vi "GraphSettings(SubVI).vi"(8 "Error In":errorcluster, 10 "XYGraph Refnum":refnum<vi>, 11 "Cluster in":refnum<vi>) -> (0 "Error Out":errorcluster)   [LabVIEW 2018]
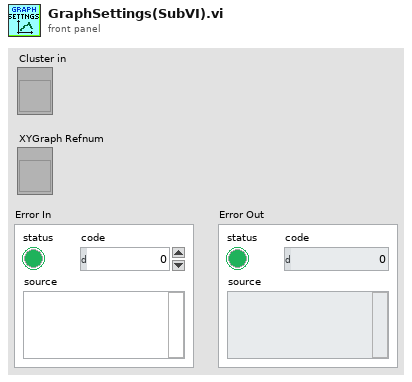
[diagram p1: front panel]
types:
  T1 = typedef "Graph settings.ctl" = cluster{"Axis X Min":dbl, "Axis X Name":string, "Axis X Max":dbl, "Axis Y Min":dbl, " Axis Y Name":string, "Axis Y Max":dbl, "Autoscale":enum16{"Yes", "No", "Only Oy", "Only Ox"}, "Choice Line":dbl}
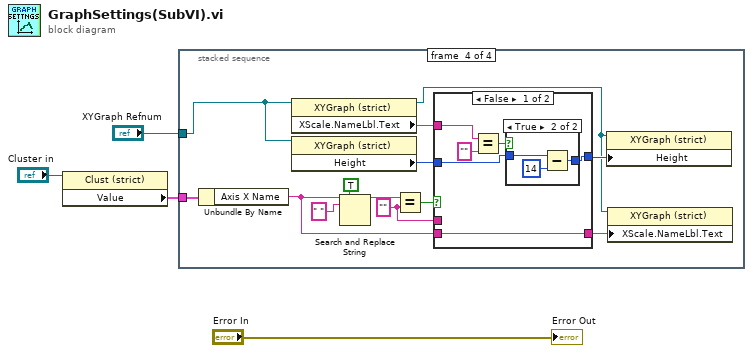
[diagram p0: block diagram]
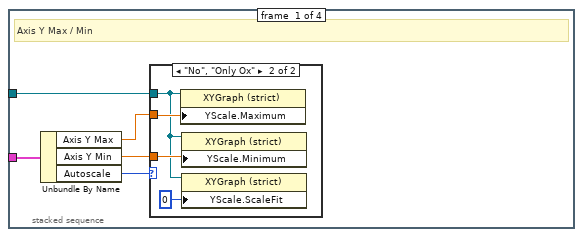
[diagram p2: hidden frame]
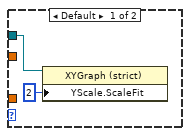
[diagram p3: hidden frame]
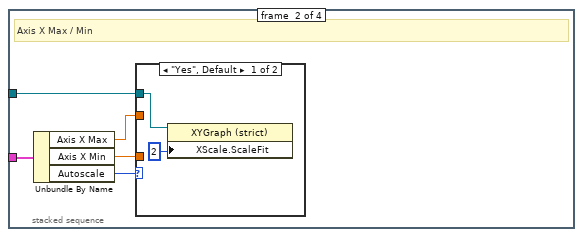
[diagram p4: hidden frame]
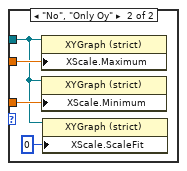
[diagram p5: hidden frame]
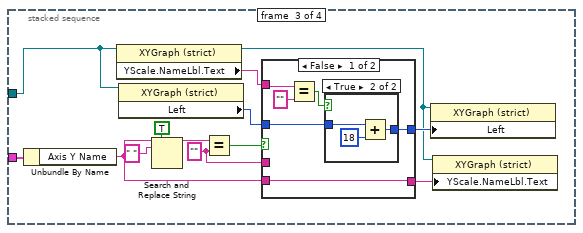
[diagram p6: hidden frame]
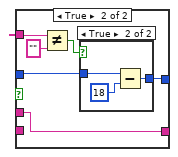
[diagram p8: hidden frame]
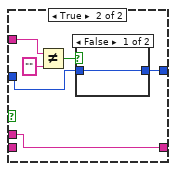
[diagram p11: hidden frame]
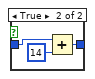
[diagram p12: hidden frame]
diagram:
  n1 = property on="Property Node" class="Clust (strict)"(reference="Cluster in") -> ("Value"=w4:T1)  [unwired: 1 in, 2 out]
  n2 = stacked-sequence {
    tunnel: w4 -> [w9 w20 w30 w63]
    tunnel: "XYGraph Refnum" -> [w5 w16 w28 w61]
    frame #0 {
      # "Axis Y Max / Min"
      n3 = Unbundle By Name(w9) -> ("Axis Y Max"=w8:dbl, "Axis Y Min"=w7:dbl, "Autoscale"=w6:enum16{"Yes", "No", "Only Oy", "Only Ox"})
      n4 = case shown="\"No\", \"Only Ox\"" w6 {
        tunnel: w8 -> [_ w15]
        tunnel: w7 -> [_ w14]
        tunnel: w5 -> [w10 w12]
        frame Default {
          n5 = property on="Property Node" class="XYGraph (strict)"(reference=w10, "YScale.ScaleFit"=u8 2 ("Y Scale.Scale Fit")) -> ()  [unwired: 1 in, 2 out]
        }
        frame "No", "Only Ox" {
          n6 = property on="Property Node" class="XYGraph (strict)"(reference=w12, "YScale.Maximum"=w15) -> ()  [unwired: 1 in, 2 out]
          n7 = property on="Property Node" class="XYGraph (strict)"(reference=w12, "YScale.Minimum"=w14) -> ()  [unwired: 1 in, 2 out]
          n8 = property on="Property Node" class="XYGraph (strict)"(reference=w12, "YScale.ScaleFit"=u8 0 ("Y Scale.Scale Fit")) -> ()  [unwired: 1 in, 2 out]
        }
      }
    }
    frame #1 {
      # "Axis X Max / Min"
      n9 = Unbundle By Name(w20) -> ("Axis X Max"=w18:dbl, "Axis X Min"=w17:dbl, "Autoscale"=w19:enum16{"Yes", "No", "Only Oy", "Only Ox"})
      n10 = case shown="\"Yes\", Default" w19 {
        tunnel: w18 -> [_ w26]
        tunnel: w17 -> [_ w25]
        tunnel: w16 -> [w21 w23]
        frame "Yes", Default {
          n11 = property on="Property Node" class="XYGraph (strict)"(reference=w21, "XScale.ScaleFit"=u8 2 ("X Scale.Scale Fit")) -> ()  [unwired: 1 in, 2 out]
        }
        frame "No", "Only Oy" {
          n12 = property on="Property Node" class="XYGraph (strict)"(reference=w23, "XScale.Maximum"=w26) -> ()  [unwired: 1 in, 2 out]
          n13 = property on="Property Node" class="XYGraph (strict)"(reference=w23, "XScale.Minimum"=w25) -> ()  [unwired: 1 in, 2 out]
          n14 = property on="Property Node" class="XYGraph (strict)"(reference=w23, "XScale.ScaleFit"=u8 0 ("X Scale.Scale Fit")) -> ()  [unwired: 1 in, 2 out]
        }
      }
    }
    frame #2 {
      w37 = "" ("y")
      n15 = Unbundle By Name(w30) -> ("Axis Y Name"=w29:string)
      n16 = property on="Property Node" class="XYGraph (strict)"(reference=w28) -> (reference out=w27:refnum<vi>, "YScale.NameLbl.Text"=w35:string)  [unwired: 1 in, 1 out]
      n17 = property on="Property Node" class="XYGraph (strict)"(reference=w28) -> ("Left"=w36:i32)  [unwired: 1 in, 2 out]
      n18 = Search and Replace String(replace all?=TRUE ("replace all? (F)"), input string=w29, search string=" ") -> (result string=w31:string)  [unwired: 5 in, 3 out]
      n19 = Equal?(x=w31, y=w37) -> (x = y?=w32:bool)
      n20 = case shown="False" w32 {
        tunnel: [w45 w55] -> w33
        tunnel: w29 -> [w45 _]
        tunnel: w37 -> [_ w55]
        tunnel: [w41 w51] -> w34
        tunnel: w35 -> [w42 w50]
        tunnel: w36 -> [w40 w52]
        frame False {
          n21 = Equal?(x=w42, y="") -> (x = y?=w44:bool)
          n22 = case shown="True" w44 {
            tunnel: [w46 w48] -> w41
            tunnel: w40 -> [w46 w47]
            frame False {
            }
            frame True {
              n23 = Add(x=w47, y=18) -> (x+y=w48:i32)
            }
          }
        }
        frame True {
          n24 = Not Equal?(x=w50, y="") -> (x != y?=w54:bool)
          n25 = case shown="True" w54 {
            tunnel: [w56 w58] -> w51
            tunnel: w52 -> [w56 w57]
            frame False {
            }
            frame True {
              n26 = Subtract(x=w57, y=18) -> (x-y=w58:i32)
            }
          }
        }
      }
      n27 = property on="Property Node" class="XYGraph (strict)"(reference=w27, "Left"=w34) -> ()  [unwired: 1 in, 2 out]
      n28 = property on="Property Node" class="XYGraph (strict)"(reference=w27, "YScale.NameLbl.Text"=w33) -> ()  [unwired: 1 in, 2 out]
    }
    frame #3 {
      w70 = "" ("y")
      n29 = Unbundle By Name(w63) -> ("Axis X Name"=w62:string)
      n30 = property on="Property Node" class="XYGraph (strict)"(reference=w61) -> (reference out=w60:refnum<vi>, "XScale.NameLbl.Text"=w66:string)  [unwired: 1 in, 1 out]
      n31 = property on="Property Node" class="XYGraph (strict)"(reference=w61) -> ("Height"=w67:u32)  [unwired: 1 in, 2 out]
      n32 = Search and Replace String(replace all?=TRUE ("replace all? (F)"), input string=w62, search string=" ") -> (result string=w64:string)  [unwired: 5 in, 3 out]
      n33 = Equal?(x=w64, y=w70) -> (x = y?=w65:bool)
      n34 = case shown="False" w65 {
        tunnel: w66 -> [w76 w85]
        tunnel: w67 -> [w75 w84]
        tunnel: [w74 w83] -> w68
        tunnel: w62 -> [w73 _]
        tunnel: [w73 w88] -> w69
        tunnel: w70 -> [_ w88]
        frame False {
          n35 = Equal?(x=w76, y="") -> (x = y?=w78:bool)
          n36 = case shown="True" w78 {
            tunnel: [w79 w81] -> w74
            tunnel: w75 -> [w79 w80]
            frame False {
            }
            frame True {
              n37 = Subtract(x=w80, y=u32 14) -> (x-y=w81:u32)
            }
          }
        }
        frame True {
          n38 = Not Equal?(x=w85, y="") -> (x != y?=w87:bool)
          n39 = case shown="False" w87 {
            tunnel: [w89 w91] -> w83
            tunnel: w84 -> [w89 w90]
            frame False {
            }
            frame True {
              n40 = Add(x=w90, y=u32 14) -> (x+y=w91:u32)
            }
          }
        }
      }
      n41 = property on="Property Node" class="XYGraph (strict)"(reference=w60, "Height"=w68) -> ()  [unwired: 1 in, 2 out]
      n42 = property on="Property Node" class="XYGraph (strict)"(reference=w60, "XScale.NameLbl.Text"=w69) -> ()  [unwired: 1 in, 2 out]
    }
  }
  "Error Out" <- "Error In"
